vi "Run Servicer.vi"() -> ()   [LabVIEW 2019, in "gRPC-servicer.lvlib" / "Servicer.lvclass"]
uses:
  Servicer.lvclass
  iService/iService.lvclass
  Servicer.lvclass/Servicer.ctl
panel:
  in  "Async [T] / Sync [F]":bool
  out "Listening Port":i32
  in  "Stop":bool
  in  "Server Address":string="localhost:50051"
  in  "Server Certificate File (.crt)":path
  in  "Server Key File (.key)":path
  # "Note: If you want the service to auto find the listening port, then enter the port number in \"Server Address\" as 0. Ex: localhost:0"
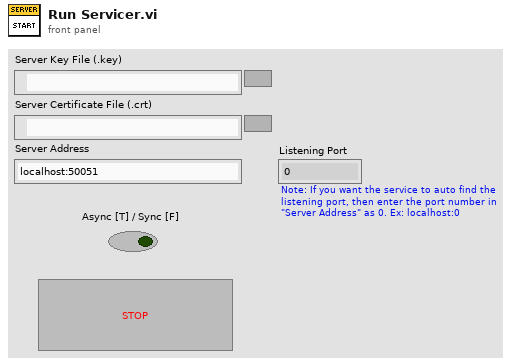
[diagram p1: front panel]
types:
  T1 = typedef "gprc-lvsupport-release.lvlib/grpcId.ctl" = u64
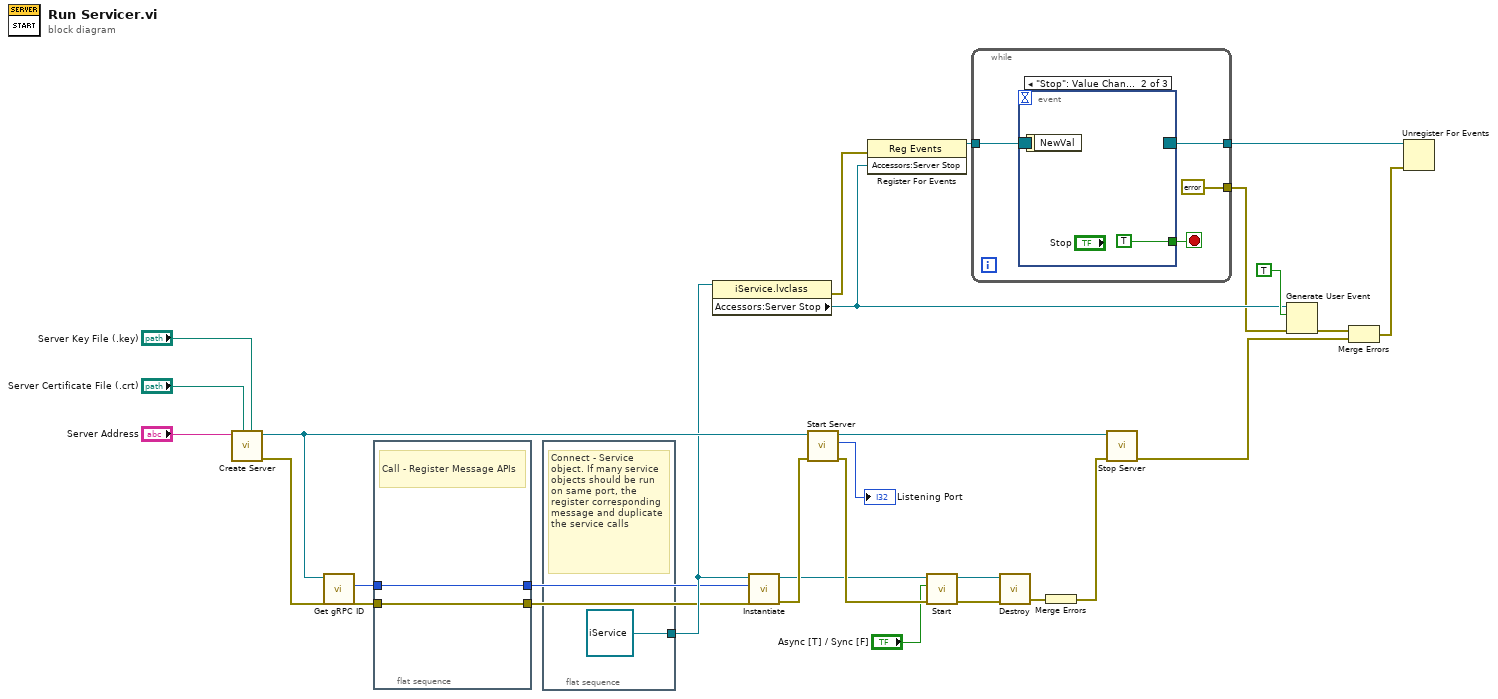
[diagram p0: block diagram]
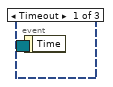
[diagram p2: hidden frame]
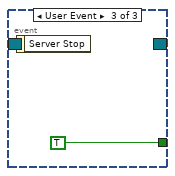
[diagram p3: hidden frame]
diagram:
  n1 = call "Create Server.vi"("Server Key File (.key)"="Server Key File (.key)", "Server Certificate File (.crt)"="Server Certificate File (.crt)", "Server Address"="Server Address") -> ("error out"=w8:errorcluster, "gRPC Server out"=w21:refnum<class "Servicer.lvclass">)  [unwired: 7 in]
  n2 = call "Get gRPC ID.vi"("OOP Server in"=w21) -> ("gRPC ID"=w9:T1)  [unwired: 9 in, 1 out]
  n3 = flat-sequence {
    tunnel: w9 -> [w29]
    tunnel: w8 -> [w30]
    tunnel: [w30] -> w7
    tunnel: [w29] -> w6
    frame #0 {
      # "Call - Register Message APIs"
    }
  }
  n4 = flat-sequence {
    tunnel: [refnum<class "iService.lvclass"> refnum ("gRPC-servicer.lvlib:iService.lvclass")] -> w10
    frame #0 {
      # "Connect - Service object. If many service objects should be run on same port, the register corresponding message and duplicate the service calls"
    }
  }
  n5 = property class="iService.lvclass"(reference=w10) -> (error out=w20:errorcluster, "Accessors:Server Stop"=w15:refnum<user-event>)  [unwired: 1 in, 1 out]
  n6 = call-dynamic "Instantiate.vi"("error in (no error)"=w7, "gRPCid"=w6, "iService"=w10) -> ("error out"=w19:errorcluster, "iService"=w3:refnum<class "iService.lvclass">)  [unwired: 7 in]
  n7 = call "Start Server.vi"("error in (no error)"=w19, "gRPC Server in"=w21) -> ("error out"=w5:errorcluster, "Listening Port"=→"Listening Port":i32, "gRPC Server out"=w28:refnum<class "Servicer.lvclass">)  [unwired: 7 in]
  n8 = register-events(error in=w20, w15) -> (reference out=w24:refnum<event-registration>)  [unwired: 1 in, 1 out]
  n9 = call-dynamic "Start.vi"("error in (no error)"=w5, "ASync [T]"="Async [T] / Sync [F]", "iService in"=w3) -> ("error out"=w4:errorcluster, "iService out"=w2:refnum<class "iService.lvclass">)  [unwired: 7 in]
  n10 = while {
    tunnel: w24 -> [w35]
    tunnel: [w33] -> w23
    tunnel: [errorcluster {"status"=FALSE, "code"=0, "source"=""} ("error constant")] -> w12
    stop <- w34 stop-if-true
    n11 = event shown="[1] \"Stop\": Value Change" {
      selector: w35 -> [_ _ _]
      dyn-events: [_ _ _] -> w33
      timeout: _ -> [_ _ _]
      tunnel: [_ TRUE TRUE] -> w34
      event Timeout {
        n12 = event-data() -> ()  [unwired: 1 in, 1 out]
      }
      event "Stop": Value Change {
        n13 = event-data() -> ()  [unwired: 1 in, 1 out]
      }
      event User Event {
        n14 = event-data() -> ()  [unwired: 1 in, 1 out]
      }
    }
  }
  n15 = call-dynamic "Destroy.vi"("error in (no error)"=w4, "SignalGeneratorService in"=w2) -> ("error out"=w18:errorcluster)  [unwired: 8 in, 1 out]
  n16 = Merge Errors(w18) -> (w17:errorcluster)
  n17 = call "Stop Server.vi"("error in (no error)"=w17, "gRPC Server in"=w28) -> ("error out"=w11:errorcluster)  [unwired: 9 in]
  n18 = Generate User Event(user event=w15, event data cluster=TRUE ("event data"), error in=w12) -> (error out=w14:errorcluster)  [unwired: 1 in, 1 out]
  n19 = Merge Errors(w14, w11) -> (w13:errorcluster)
  n20 = Unregister For Events(event registration refnum=w23, error in=w13) -> ()  [unwired: 1 out]
